vi "ShowExperimentWindow.vi"(9 "AvailableExperiments":T1[](array[typedef]), 10 "Value":u16, 11 "Value 2":i32) -> ()   [LabVIEW 2017]
uses:
  Types/ExperimentGrp.ctl
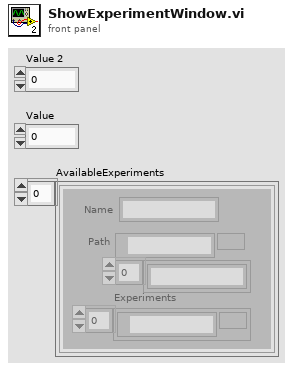
[diagram p1: front panel]
types:
  T1 = typedef "ExperimentGrp.ctl" = cluster{"Path":path, "Experiments":path[], "Name":string, "Experiment Names":string[]}
  T2 = enum32{"Bad", "Idle", "Run top level", "Running"}
  T3 = enum32{"Invalid", "Standard", "Closed", "Hidden", "Minimized", "Maximized"}
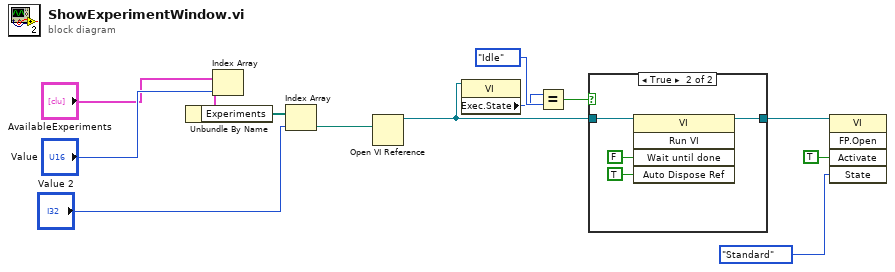
[diagram p0: block diagram]
diagram:
  n1 = Index Array(array="AvailableExperiments", index="Value") -> (element=w2:T1)
  n2 = Unbundle By Name(w2) -> ("Experiments"=w3:path[])
  n3 = Index Array(array=w3, index="Value 2") -> (element=w6:path)
  n4 = Open VI Reference(vi path=w6) -> (vi reference=w10:refnum<vi>)  [unwired: 5 in, 1 out]
  n5 = property class="VI"(reference=w10) -> ("Exec.State"=w12:T2)  [unwired: 1 in, 2 out]
  n6 = Equal?(x=w12, y=T2."Idle" ("Execution:State")) -> (x = y?=w11:bool)
  n7 = case shown="True" w11 {
    tunnel: [w14 w16] -> w9
    tunnel: w10 -> [w14 w15]
    frame False {
    }
    frame True {
      n8 = invoke class="VI" method="Run VI"(reference=w15, "Wait until done"=FALSE ("Wait Until Done"), "Auto Dispose Ref"=TRUE ("Auto Dispose Reference")) -> (reference out=w16:refnum<vi>)  [unwired: 2 in, 4 out]
    }
  }
  n9 = invoke class="VI" method="FP.Open"(reference=w9, "Activate"=TRUE ("Activate?"), "State"=T3."Standard") -> ()  [unwired: 2 in, 5 out]
